vi "TH_MeanVal.vi"(2 "NewValues In":bool[](array[boolean]), 3 "Humidities In":dbl[](array[numeric]) format="%.2f", 4 "Temperatures In":dbl[](array[numeric]) format="%.2f", 5 "MeanTime (sec)":dbl format="%.2f") -> (0 "MeanHum":dbl[](array[numeric]) format="%.2f", 1 "MeanTemp":dbl[](array[numeric]) format="%.2f")   [LabVIEW 2014]
uses:
  TH_Globals.vi
panel:
  out "StartTime":dbl format="%.2f"
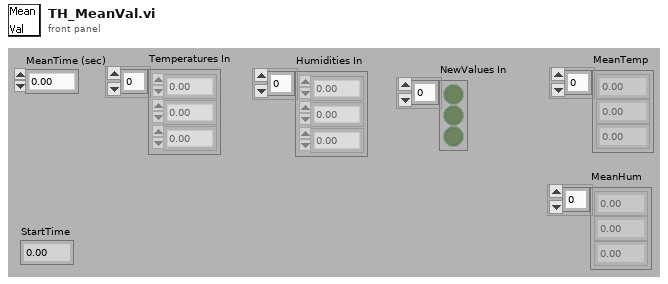
[diagram p1: front panel]
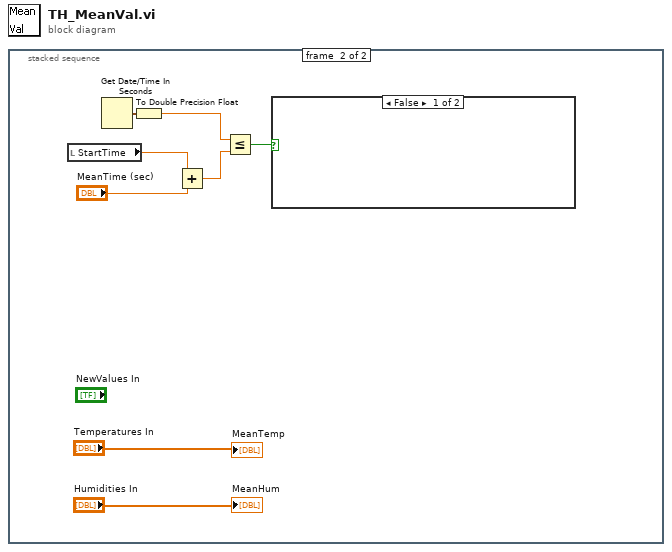
[diagram p0: block diagram]
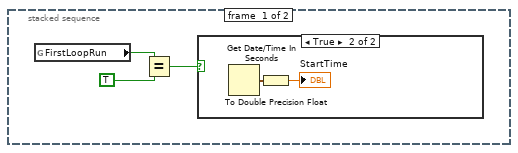
[diagram p2: hidden frame]
diagram:
  n1 = stacked-sequence {
    frame #0 {
      n2 = global read "TH_Globals.vi" "FirstLoopRun"() -> (w3:bool)
      n3 = Equal?(x=w3, y=TRUE) -> (x = y?=w1:bool)
      n4 = case shown="True" w1 {
        frame False {
        }
        frame True {
          n5 = Get Date/Time In Seconds() -> (seconds since 1Jan1904=w4:timestamp)
          n6 = To Double Precision Float(number=w4) -> (double precision float=→"StartTime":dbl)
        }
      }
    }
    frame #1 {
      n7 = local read "StartTime"() -> (w12:dbl)
      n8 = Get Date/Time In Seconds() -> (seconds since 1Jan1904=w6:timestamp)
      n9 = To Double Precision Float(number=w6) -> (double precision float=w13:dbl)
      n10 = Add(x=w12, y="MeanTime (sec)") -> (x+y=w10:dbl)
      n11 = Less Or Equal?(x=w13, y=w10) -> (x <= y?=w9:bool)
      n12 = case shown="False" w9 {
        frame False {
        }
        frame True {
        }
      }
      "MeanTemp" <- "Temperatures In"
      "MeanHum" <- "Humidities In"
    }
  }
